vi "FIFO Check.vi"(0 "FPGA Ref in":T3, 5 "Read at least # points":u32, 7 "Imaging Protocol":T1, 11 "error in (no error)":errorcluster) -> (4 "FPGA Ref out":T3, 6 "Elements Available":T2, 8 "Both channels no more data (delayed by 1 iteration)":bool, 10 "Data available or data has just completed (read the FIFO)":bool, 15 "error out":errorcluster)   [LabVIEW 2017]
uses:
  RIG-SPECIFIC FILES/FPGA Refs/FPGA Ref.ctl
  Acquisition/Typedefs/FIFO elements available.ctl
  Typedefs/Imaging Protocols enum.ctl
  <vilib>/Utility/error.llb/Error Cluster From Error Code.vi
  <vilib>/rvi/errors/niLvFpgaAdjustHostInterfaceError.vi
  <vilib>/rvi/interface/nirviMethod/nirviMethod.xnode
  <vilib>/rvi/errors/niLvFpgaMergeErrorWithErrorCode.vi
  <vilib>/FPGAPlugInAG/Dynamic/niLvFpga_ReadFifo_Dynamic.vi
panel:
  out "No more data Ch1":bool
  out "No more data Ch0":bool
  out "Registered peak value":dbl
  in  "Timeout (ms)":i32=30
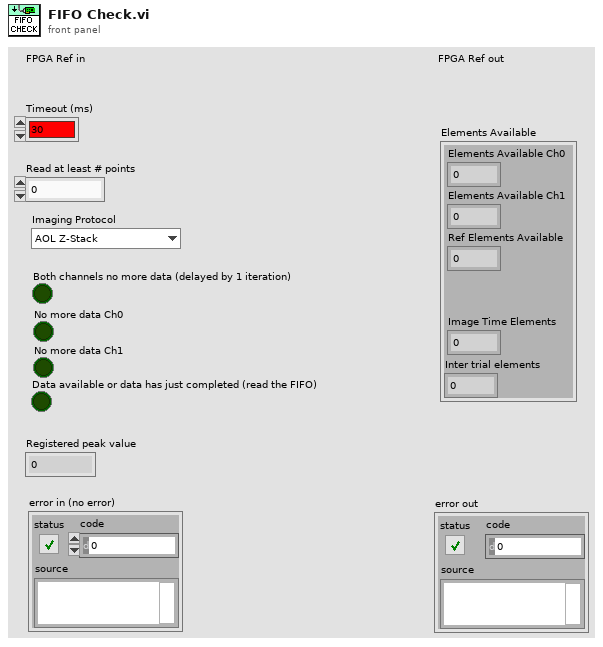
[diagram p1: front panel]
types:
  T1 = typedef "Imaging Protocols enum.ctl" = enum16{"AOL Z-Stack", "Motor Z Stack", "Functional Acquisition", "Single Plane Acquisition", "Volume Acquisition", "Live Imaging", "Live Plane Imaging", "Live Volume Imaging"}
  T2 = typedef "FIFO elements available.ctl" = cluster{"Elements Available Ch0":u32, "Elements Available Ch1":u32, "Ref Elements Available":u32, "Image Time Elements":u32, "Inter trial elements":u32}
  T3 = typedef "FPGA Ref.ctl" = refnum<k20>
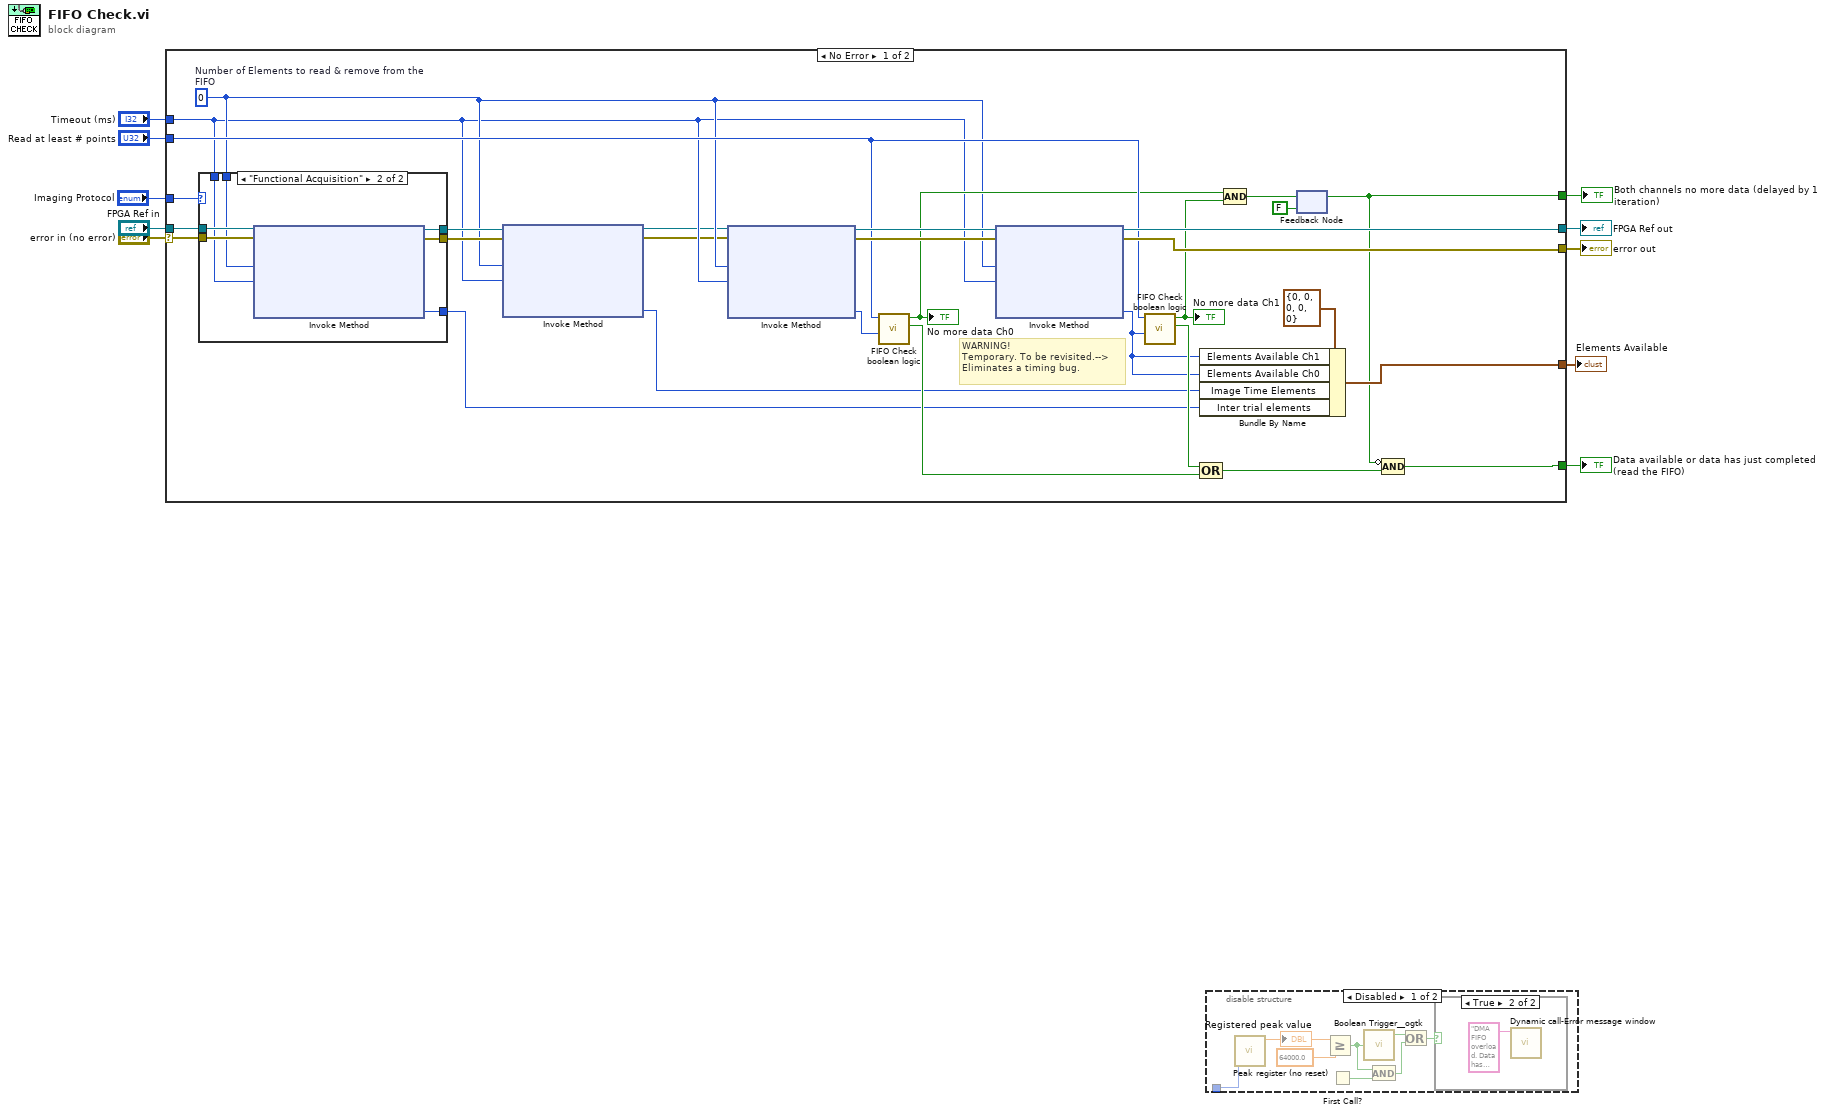
[diagram p0: block diagram]
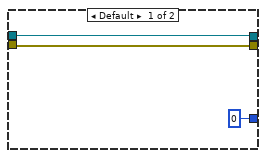
[diagram p2: hidden frame]
diagram:
  n1 = case shown="No Error" "error in (no error)" {
    selector: "error in (no error)" -> [w19 w51]
    tunnel: [w24 _] -> w10
    tunnel: [w39 w50] -> w9
    tunnel: "FPGA Ref in" -> [w20 w50]
    tunnel: "Timeout (ms)" -> [w15 _]
    tunnel: [w36 w51] -> w6
    tunnel: "Read at least # points" -> [w35 _]
    tunnel: [w33 _] -> w2
    tunnel: [w23 _] -> w3
    tunnel: "Imaging Protocol" -> [w13 _]
    frame No Error {
      w16 = u32 0  # Number of Elements to read & remove from the FIFO
      # "WARNING!\nTemporary. To be revisited.-->\nEliminates a timing bug."
      n2 = case shown="\"Functional Acquisition\"" w13 {
        tunnel: w20 -> [w42 w49]
        tunnel: w19 -> [w41 w48]
        tunnel: [w42 w47] -> w18
        tunnel: [w41 w46] -> w17
        tunnel: w16 -> [_ w45]
        tunnel: w15 -> [_ w44]
        tunnel: [u32 0 ("Elements Remaining") w43] -> w14
        frame Default {
        }
        frame "Functional Acquisition" {
          n3 = xnode ("Invoke Method")("FPGA VI Reference In"=w49, "error in"=w48, "Number of Elements"=w45, "Timeout (ms)"=w44) -> ("FPGA VI Reference Out"=w47:T3, "error out"=w46:errorcluster, "Elements Remaining"=w43:u32)  [unwired: 1 out]
        }
      }
      n4 = xnode ("Invoke Method")("FPGA VI Reference In"=w18, "error in"=w17, "Number of Elements"=w16, "Timeout (ms)"=w15) -> ("FPGA VI Reference Out"=w11:T3, "error out"=w12:errorcluster, "Elements Remaining"=w21:u32)  [unwired: 1 out]
      n5 = xnode ("Invoke Method")("FPGA VI Reference In"=w11, "error in"=w12, "Number of Elements"=w16, "Timeout (ms)"=w15) -> ("FPGA VI Reference Out"=w38:T3, "error out"=w37:errorcluster, "Elements Remaining"=w31:u32)  [unwired: 1 out]
      n6 = call "FIFO Check boolean logic.vi"("Elements Remaining"=w31, "Read at least"=w35) -> ("Read FIFO"=w32:bool, "No more data"=w29:bool)  [unwired: 8 in]
      "No more data Ch0" <- w29
      n7 = xnode ("Invoke Method")("FPGA VI Reference In"=w38, "error in"=w37, "Number of Elements"=w16, "Timeout (ms)"=w15) -> ("FPGA VI Reference Out"=w39:T3, "error out"=w36:errorcluster, "Elements Remaining"=w30:u32)  [unwired: 1 out]
      n8 = call "FIFO Check boolean logic.vi"("Elements Remaining"=w30, "Read at least"=w35) -> ("Read FIFO"=w34:bool, "No more data"=w28:bool)  [unwired: 8 in]
      "No more data Ch1" <- w28
      n9 = Bundle By Name(cluster=T2 {"Elements Available Ch0"=0, "Elements Available Ch1"=0, "Ref Elements Available"=0, "Image Time Elements"=0, "Inter trial elements"=0} ("Elements Available 2"), "Elements Available Ch1"=w30, "Elements Available Ch0"=w30, "Image Time Elements"=w21, "Inter trial elements"=w14) -> (w33:T2)
      n10 = Compound Arithmetic op=OR(w34, w32) -> (w25:bool)
      n11 = Compound Arithmetic op=AND(w29, w28) -> (w27:bool)
      n12 = feedback-in #1(w27) -> ()
      n13 = feedback #1(FALSE) -> (w23:bool)
      n14 = Compound Arithmetic op=AND(invert w23, w25) -> (w24:bool)
    }
    frame Error {
    }
  }
  "error out" <- w6
  "FPGA Ref out" <- w9
  "Data available or data has just completed (read the FIFO)" <- w10
  "Both channels no more data (delayed by 1 iteration)" <- w3
  "Elements Available" <- w2
  n15 = disable-structure "Diagram Disable Structure" shown="Disabled" {
    disable-tunnel: _ -> [w59 _]
    frame Disabled {
      n16 = call <userlib>:"Peak register (no reset).vi"("Value in"=w59) -> ("Registered peak value"=w58:dbl)  [unwired: 10 in]
      "Registered peak value" <- w58
      n17 = Greater Or Equal?(x=w58, y=64000.0) -> (x >= y?=w56:bool)
      n18 = First Call?() -> (First Call?: T/F=w55:bool)
      n19 = call <userlib>:"Boolean Trigger__ogtk.vi"("Boolean Input"=w56) -> ("Rising Edge"=w54:bool)  [unwired: 1 in, 1 out]
      n20 = And(x=w56, y=w55) -> (x .and. y?=w53:bool)
      n21 = Or(x=w54, y=w53) -> (x .or. y?=w52:bool)
      n22 = case shown="True" w52 {
        frame False {
        }
        frame True {
          n23 = call "Dynamic call-Error message window.vi"("Error Message"="DMA FIFO overload. Data has been lost.") -> ()  [unwired: 10 in, 1 out]
        }
      }
    }
    frame Enabled {
    }
  }
